vi "AlarmExportTrendToSpreadsheetRequest_Name.vi"() -> (1 "MessageName":string)   [LabVIEW 2017]
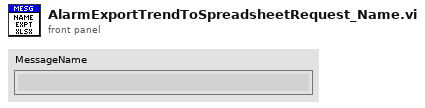
[diagram p1: front panel]
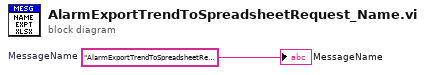
[diagram p0: block diagram]
diagram:
  w1 = "AlarmExportTrendToSpreadsheetRequest"  # MessageName
  "MessageName" <- w1
